vi "Create Coverage Report - No Project Files - Reports No Packages.vi"() -> ()   [LabVIEW 2017, in "Cobertura.Tests.lvlib"]
uses:
  Cobertura.Tests.lvlib
  Fake Code Coverage/Fake Code Coverage.lvclass
  C:/Users/pasca/Projects/Home/lvunit/CodeCoverage/CodeCoverage.lvclass
  Fake Code Inspector/Fake Code Inspector.lvclass
  C:/Users/pasca/Projects/Home/lvunit/Cobertura/Code Inspector Base/Code Inspector Base.lvclass
  Fake Project Inspector/Fake Project Inspector.lvclass
  C:/Users/pasca/Projects/Home/lvunit/Cobertura/Project Inspector Base/Project Inspector Base.lvclass
  Cobertura/Coverage/Coverage.lvclass/Coverage.ctl
  Cobertura/Coverage/Read Packages.vi
  Cobertura/Package/Package.lvclass
  Cobertura/Cobertura.lvlib
  Cobertura/Coverage/Coverage.lvclass
  <vilib>/PNR/Transparent Assertions/Transparent Assertions/Transparent Assertions.lvlib
panel:
  out "error out":errorcluster
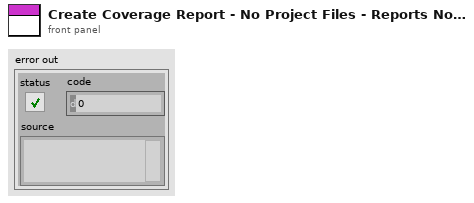
[diagram p1: front panel]
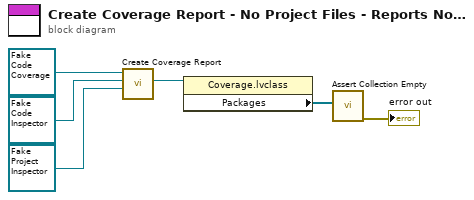
[diagram p0: block diagram]
diagram:
  n1 = call "Create Coverage Report.vi"("Project Inspector"=refnum<class "Fake Project Inspector.lvclass"> refnum ("Cobertura.Tests.lvlib:Fake Project Inspector.lvclass"), "Code Inspector"=refnum<class "Fake Code Inspector.lvclass"> refnum ("Cobertura.Tests.lvlib:Fake Code Inspector.lvclass"), "CodeCoverage in"=refnum<class "Fake Code Coverage.lvclass"> refnum ("Cobertura.Tests.lvlib:Fake Code Coverage.lvclass")) -> ("Coverage"=w6:refnum<class "Coverage.lvclass">)  [unwired: 7 in, 1 out]
  n2 = property class="Coverage.lvclass"(reference=w6) -> ("Packages"=w4:refnum<class "Package.lvclass">[])  [unwired: 1 in, 2 out]
  n3 = call <vilib>:"Assert Collection Empty.vi"("Collection"=w4) -> ("error out"=→"error out":errorcluster)  [unwired: 10 in]
